vi "SQL Fetch Data.vi"(8 "error in (no error)":errorcluster, 11 "ADODB._Recordset In":refnum<k7>) -> (0 "error out":errorcluster, 1 "ADODB._Recordset Out":refnum<k7>, 2 "Rows Fetched":i32, 3 "Data":string[][](array[string]))   [LabVIEW 2013]
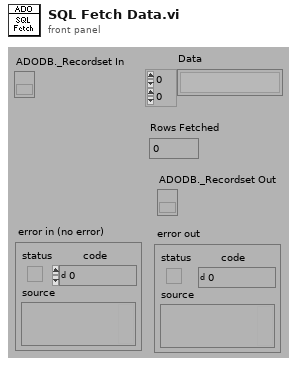
[diagram p1: front panel]
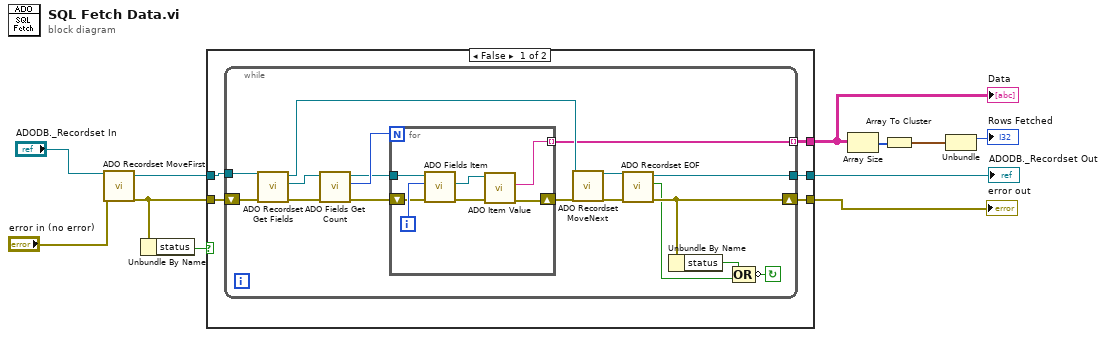
[diagram p0: block diagram]
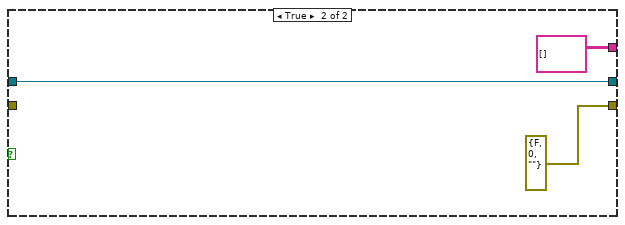
[diagram p2: hidden frame]
diagram:
  n1 = call "ADO Recordset MoveFirst.vi"("ADODB._Recordset In"="ADODB._Recordset In", "error in (no error)"="error in (no error)") -> ("ADODB._Recordset Out"=w11:refnum<k7>, "error out"=w6:errorcluster)  [unwired: 16 in]
  n2 = Unbundle By Name(w6) -> ("status"=w5:bool)
  n3 = case shown="False" w5 {
    tunnel: w6 -> [w16 _]
    tunnel: w11 -> [w15 w41]
    tunnel: [w14 errorcluster {"status"=FALSE, "code"=0, "source"=""} ("error out")] -> w2
    tunnel: [w13 string[][] []] -> w10
    tunnel: [w12 w41] -> w1
    frame False {
      n4 = while {
        shift-right: [w21] -> w14
        shift-left: w16 -> [w31]
        tunnel: w15 -> [w33]
        tunnel: [w22] -> w12
        tunnel: [w17] -> w13 mode=indexing
        stop <- w18 continue-if-true
        n5 = call "ADO Recordset Get Fields.vi"("error in (no error)"=w31, "ADODB._Recordset In"=w33) -> ("error out"=w30:errorcluster, "Fields Out"=w32:refnum<k7>, "ADODB._Recordset Out"=w25:refnum<k7>)  [unwired: 7 in]
        n6 = call "ADO Fields Get Count.vi"("error in (no error)"=w30, "Fields In"=w32) -> ("error out"=w27:errorcluster, "Count"=w29:i32, "Fields Out"=w28:refnum<k7>)  [unwired: 7 in]
        n7 = for {
          N: w29 -> [_]
          tunnel: w28 -> [w40]
          shift-right: [w36] -> w26
          shift-left: w27 -> [w37]
          tunnel: [w35] -> w17 mode=indexing
          i -> [w39]
          n8 = call "ADO Fields Item.vi"("error in (no error)"=w37, "Index"=w39, "Fields In"=w40) -> ("error out"=w38:errorcluster, "Item Out"=w34:refnum<k7>)  [unwired: 6 in, 1 out]
          n9 = call "ADO Item Value.vi"("error in (no error)"=w38, "Item In"=w34) -> ("error out"=w36:errorcluster, "Value"=w35:string)  [unwired: 7 in, 1 out]
        }
        n10 = call "ADO Recordset MoveNext.vi"("ADODB._Recordset In"=w25, "error in (no error)"=w26) -> ("ADODB._Recordset Out"=w23:refnum<k7>, "error out"=w24:errorcluster)  [unwired: 16 in]
        n11 = call "ADO Recordset EOF.vi"("error in (no error)"=w24, "ADODB._Recordset In"=w23) -> ("error out"=w21:errorcluster, "EOF"=w20:bool, "ADODB._Recordset Out"=w22:refnum<k7>)  [unwired: 7 in]
        n12 = Unbundle By Name(w21) -> ("status"=w19:bool)
        n13 = Compound Arithmetic op=OR(w19, w20) -> (invert w18:bool)
      }
    }
    frame True {
    }
  }
  "Data" <- w10
  "error out" <- w2
  "ADODB._Recordset Out" <- w1
  n14 = Array Size(array=w10) -> (size(s)=w9:i32[])
  n15 = Array To Cluster(array=w9) -> (cluster=w8:cluster{"[0]":i32, "[1]":i32})
  n16 = Unbundle(w8) -> ("[0]"=→"Rows Fetched":i32)  [unwired: 1 out]
